vi "test16-LosslessRegisterStatusMultipleTimesNonCSM.vi"(8 "error in (no error)":errorcluster, 11 "TestCase in":refnum<class "testcase-CSMBroadcast.lvclass">) -> (0 "error out":errorcluster, 3 "TestCase out":refnum<class "testcase-CSMBroadcast.lvclass">)   [LabVIEW 2017, in "testcase-CSMBroadcast.lvclass"]
uses:
  testcase-CSMBroadcast.lvclass
  <vilib>/addons/_JKI Toolkits/VI Tester/TestCase.llb/TestCase.lvclass
  src/user.lib/_NEVSTOP/Communicable State Machine(CSM)/Communicable State Machine.lvlib
  CSM/CSM-Testcase.lvlib
  C:/Program Files (x86)/National Instruments/LabVIEW 2017/vi.lib/addons/_JKI Toolkits/VI Tester/TestCase.llb/TestCase.lvclass
panel:
  out "Arguments":string
  out "ModuleName":string
  out "LoopCount":i32
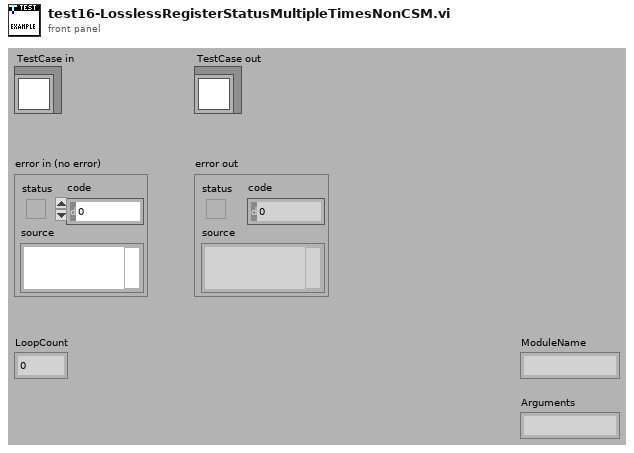
[diagram p1: front panel]
types:
  T1 = cluster{"ModuleName":string, "Status":string, "Arguments":string}
  T2 = cluster{"cluster":cluster{"ModuleName":string, "Status":string, "Arguments":string}, "Counter":u32}
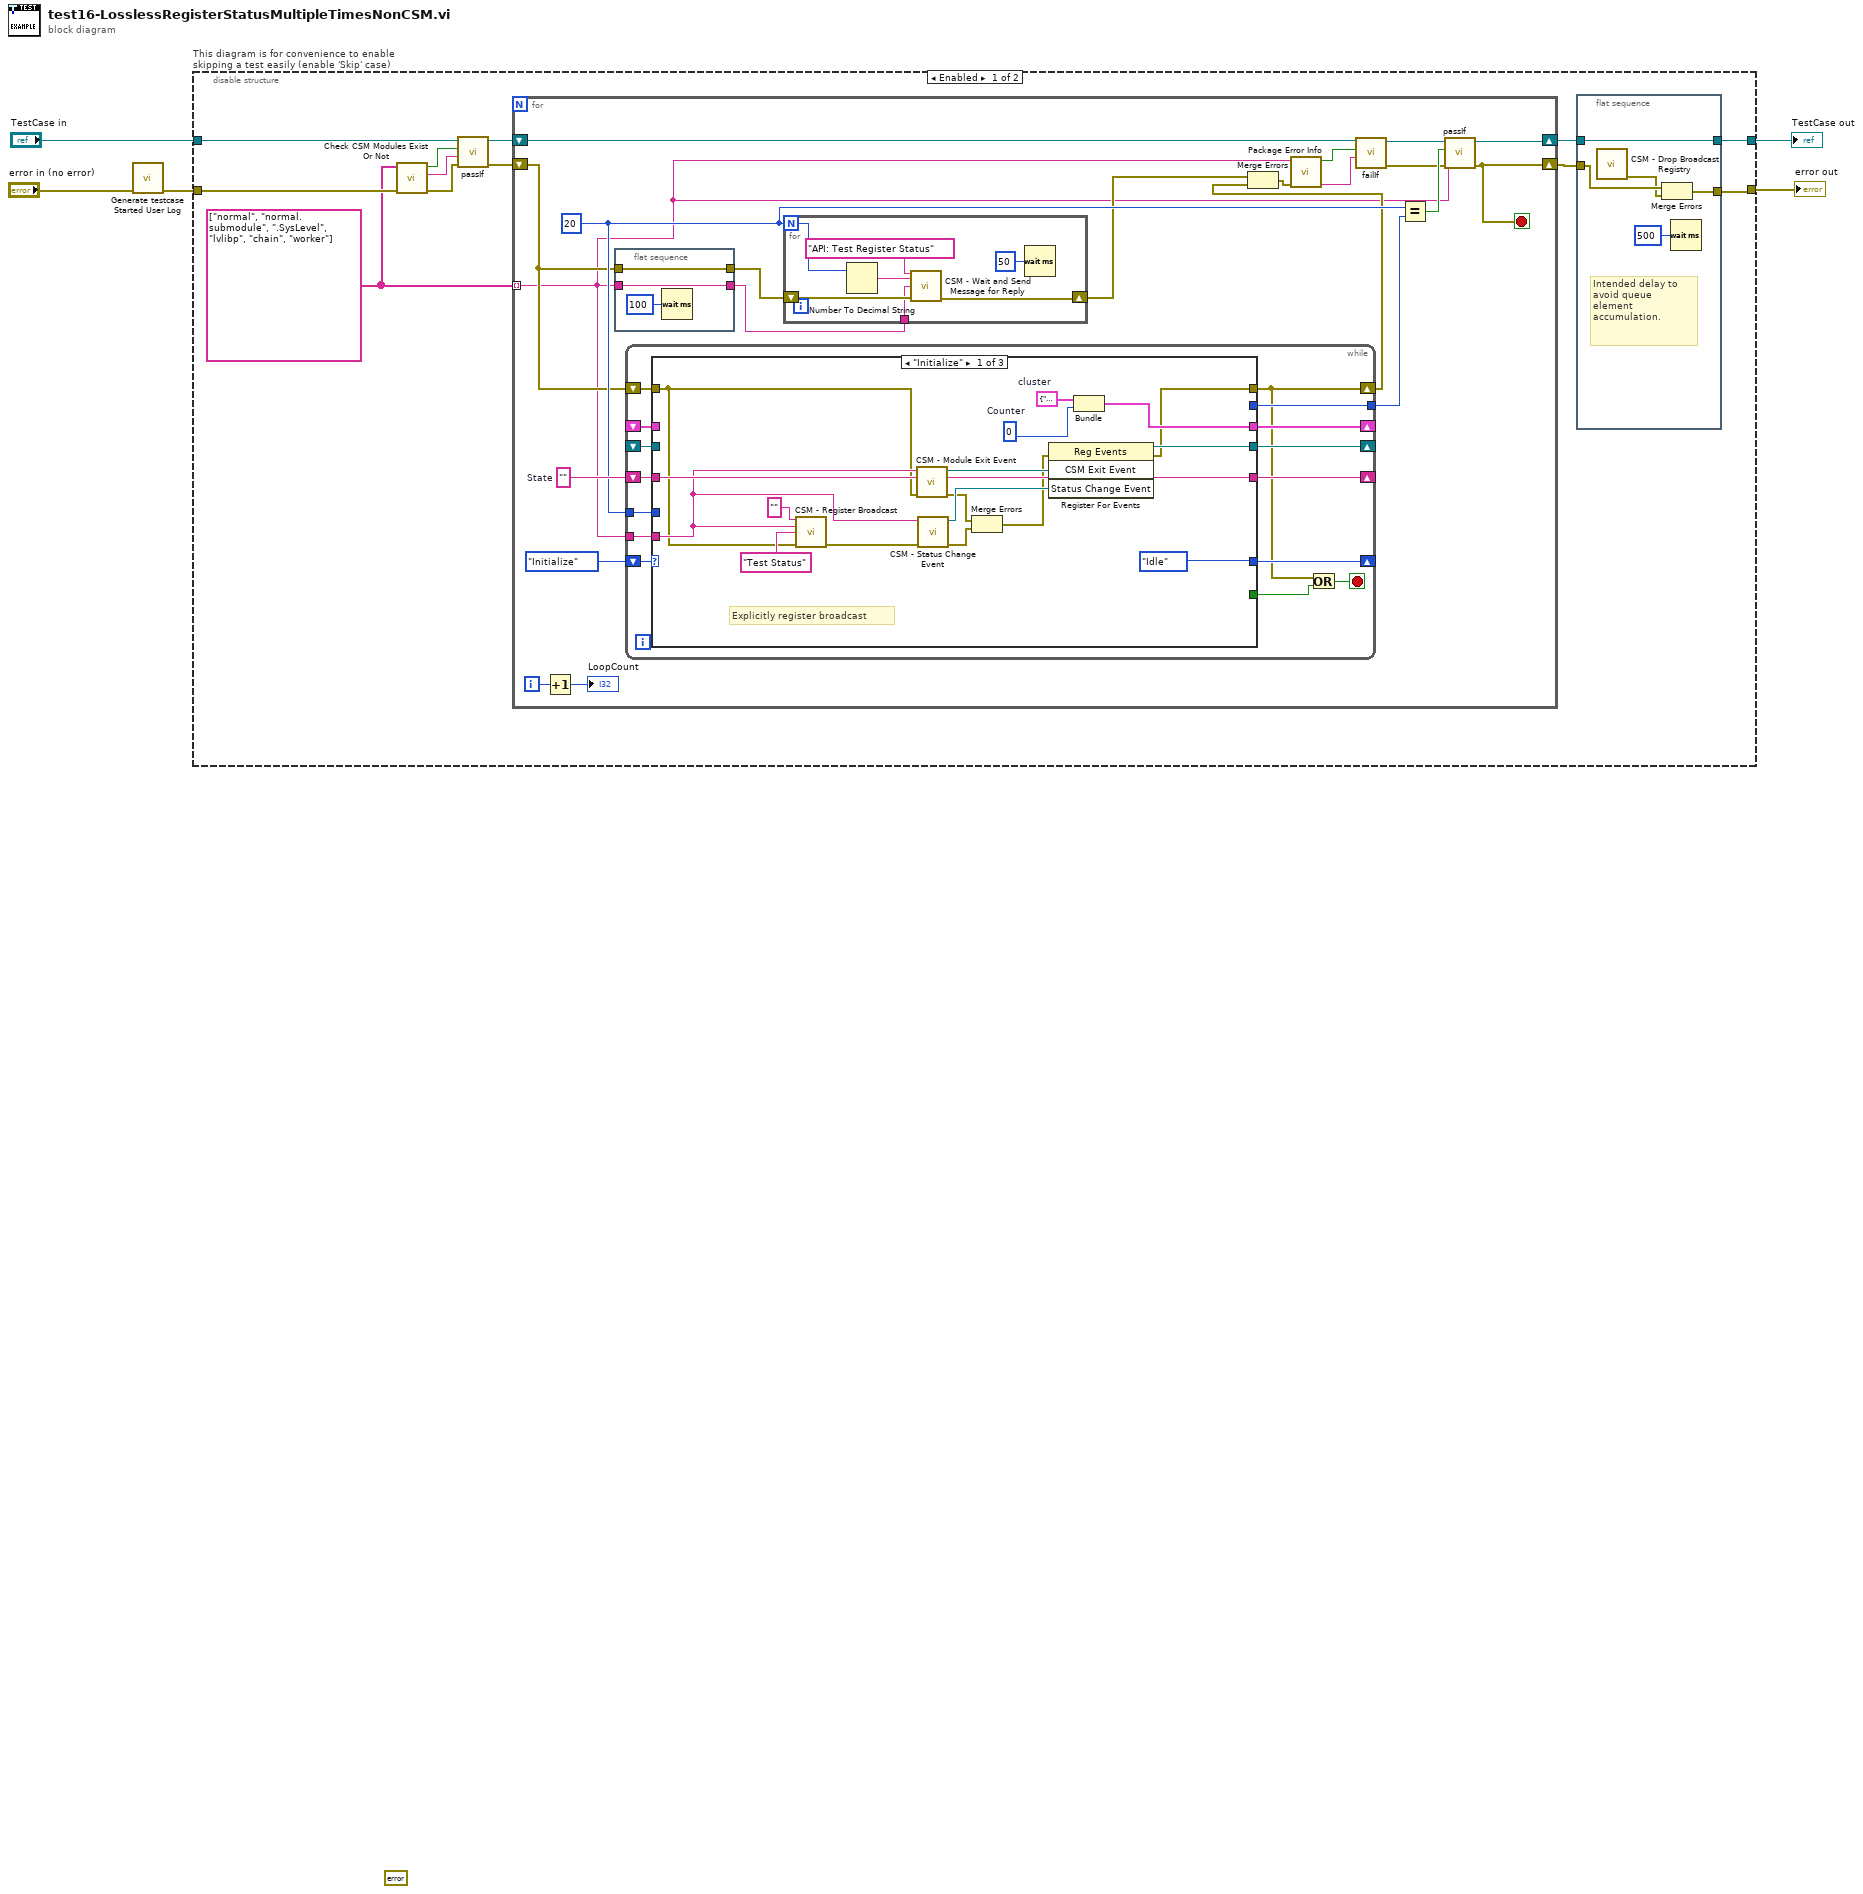
[diagram p0: block diagram]
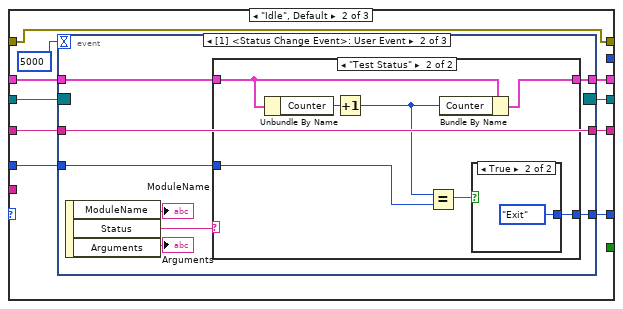
[diagram p2: hidden frame]
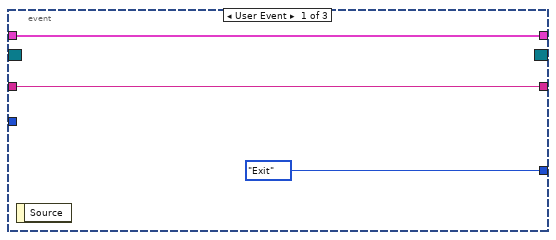
[diagram p3: hidden frame]
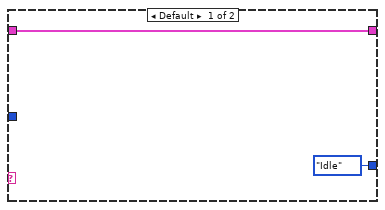
[diagram p4: hidden frame]
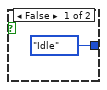
[diagram p5: hidden frame]
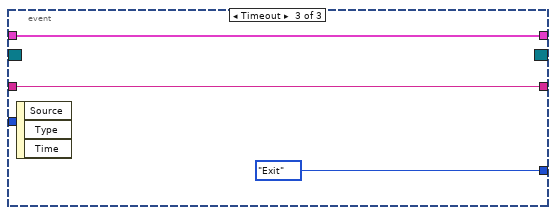
[diagram p6: hidden frame]
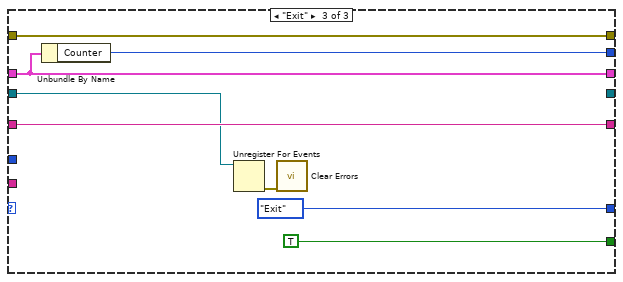
[diagram p7: hidden frame]
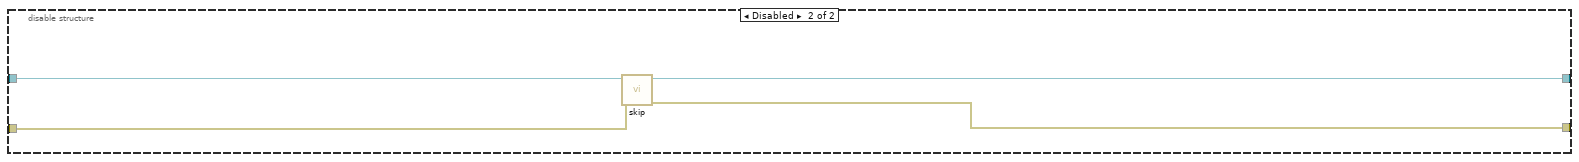
[diagram p8: hidden frame]
diagram:
  (unwired) errorcluster {"status"=FALSE, "code"=0, "source"=""} ("error out")
  n1 = call "Generate testcase Started User Log.vi"("Error In"="error in (no error)") -> ("error out"=w1:errorcluster)  [unwired: 10 in]
  n2 = disable-structure "This diagram is for convenience to enable skipping a test easily (enable 'Skip' case)" shown="Enabled" {
    disable-tunnel: "TestCase in" -> [w12 w132]
    disable-tunnel: [w6 w130] -> w3
    disable-tunnel: [w16 w131] -> w2
    disable-tunnel: w1 -> [w9 w129]
    frame Enabled {
      w8 = string[] ["normal", "normal.submodule", ".SysLevel", "lvlibp", "chain", "worker"]
      n3 = call "Check CSM Modules Exist Or Not.vi"("error in"=w9, "CSM names in"=w8) -> ("error out"=w13:errorcluster, "Debug string"=w14:string, "All Modules Exist?"=w15:bool)  [unwired: 7 in]
      n4 = call-dynamic "passIf.vi"("error in (no error)"=w13, "message (\"\")"=w14, "pass"=w15, "TestCase in"=w12) -> ("error out"=w10:errorcluster, "TestCase out"=w11:refnum<class "testcase-CSMBroadcast.lvclass">)  [unwired: 6 in]
      n5 = for {
        shift-right: [w41] -> w7
        shift-left: w11 -> [w25]
        shift-right: [w38] -> w17
        shift-left: w10 -> [w32]
        tunnel: w8 -> [w26] mode=indexing
        i -> [w40]
        stop <- w38 stop-if-true
        w34 = 20
        w42 = ""  # State
        n6 = Increment(x=w40) -> (x+1=→"LoopCount":i32)
        n7 = flat-sequence {
          tunnel: w26 -> [w53]
          tunnel: [w53] -> w37
          tunnel: w32 -> [w51]
          tunnel: [w51] -> w33
          frame #0 {
            n8 = Wait (ms)(milliseconds to wait=u32 100) -> ()  [unwired: 1 out]
          }
        }
        n9 = while {
          shift-right: [w67] -> _
          shift-left: enum16{"Idle", "Initialize", "Exit"}."Initialize" -> [w68]
          shift-right: [w65] -> _
          shift-left: w42 -> [w66]
          shift-right: [w64] -> _
          shift-left: _ -> [w63]
          shift-right: [w62] -> _
          shift-left: _ -> [w61]
          tunnel: w26 -> [w60]
          tunnel: [w59] -> w36
          tunnel: w34 -> [w58]
          shift-right: [w56] -> w29
          shift-left: w32 -> [w57]
          stop <- w54 stop-if-true
          n10 = case shown="\"Initialize\"" w68 {
            tunnel: [enum16{"Idle", "Initialize", "Exit"}."Idle" w95 enum16{"Idle", "Initialize", "Exit"}."Exit"] -> w67
            tunnel: [_ _ TRUE] -> w55
            tunnel: w66 -> [w84 w93 w126]
            tunnel: [w84 w94 w126] -> w65
            tunnel: [w82 w91 _] -> w64
            tunnel: w63 -> [_ w92 w125]
            tunnel: [w81 w89 w122] -> w62
            tunnel: w61 -> [_ w90 w122]
            tunnel: w60 -> [w73 _ _]
            tunnel: [_ _ w123] -> w59
            tunnel: w58 -> [_ w87 _]
            tunnel: w57 -> [w71 w86 w121]
            tunnel: [w69 w86 w121] -> w56
            frame "Initialize" {
              w76 = u32 0  # Counter
              w79 = T1 {"ModuleName"="", "Status"="", "Arguments"=""}  # cluster
              # "Explicitly register broadcast"
              n11 = call "CSM - Register Broadcast.vi"("CSM Name(Empty for Broadcast Event)"="", "Source CSM Name (* as Default)"=w73, "Trigger"="Test Status" ("State"), "Error In"=w71) -> ("error out"=w72:errorcluster)  [unwired: 10 in, 1 out]
              n12 = call "CSM - Module Exit Event.vi"("Error In"=w71, "Name (\"\" to Use UUID) In"=w73) -> ("error out"=w78:errorcluster, "CSM Exit Event"=w83:refnum<user-event>)  [unwired: 7 in, 1 out]
              n13 = call "CSM - Status Change Event.vi"("Error In"=w72, "CSM Module"=w73) -> ("error out"=w77:errorcluster, "Status Change Event"=w80:refnum<user-event>)  [unwired: 7 in, 1 out]
              n14 = Merge Errors(w78, w77) -> (w70:errorcluster)
              n15 = register-events(error in=w70, w83, w80) -> (reference out=w82:refnum<event-registration>, error out=w69:errorcluster)  [unwired: 1 in]
              n16 = Bundle("cluster"=w79, "Counter"=w76) -> (w81:T2)  [unwired: 1 in]
            }
            frame "Idle", Default {
              n17 = event shown="[1] <Status Change Event>: User Event" {
                selector: w92 -> [_ _ _]
                dyn-events: [_ _ _] -> w91
                timeout: 5000 -> [_ _ _]
                tunnel: [enum16{"Idle", "Initialize", "Exit"}."Exit" w105 enum16{"Idle", "Initialize", "Exit"}."Exit"] -> w95
                tunnel: w93 -> [w98 w106 w120]
                tunnel: [w98 w106 w120] -> w94
                tunnel: w90 -> [w96 w103 w119]
                tunnel: [w96 w104 w119] -> w89
                tunnel: w87 -> [_ w102 _]
                event User Event {
                  n18 = event-data() -> ()  [unwired: 1 in, 1 out]
                }
                event User Event {
                  n19 = event-data() -> ("ModuleName"=→"ModuleName":string, "Status"=w101:string, "Arguments"=→"Arguments":string)  [unwired: 1 in]
                  n20 = case shown="\"Test Status\"" w101 {
                    tunnel: [enum16{"Idle", "Initialize", "Exit"}."Idle" w115] -> w105
                    tunnel: [w108 w114] -> w104
                    tunnel: w103 -> [w108 w113]
                    tunnel: w102 -> [_ w109]
                    frame Default {
                    }
                    frame "Test Status" {
                      n21 = Unbundle By Name(w113) -> ("Counter"=w112:u32)
                      n22 = Increment(x=w112) -> (x+1=w110:u32)
                      n23 = Equal?(x=w110, y=w109) -> (x = y?=w111:bool)
                      n24 = Bundle By Name(cluster=w113, "Counter"=w110) -> (w114:T2)
                      n25 = case shown="True" w111 {
                        tunnel: [enum16{"Idle", "Initialize", "Exit"}."Idle" enum16{"Idle", "Initialize", "Exit"}."Exit"] -> w115
                        frame False {
                        }
                        frame True {
                        }
                      }
                    }
                  }
                }
                event Timeout {
                  n26 = event-data() -> ()  [unwired: 1 in, 3 out]
                }
              }
            }
            frame "Exit" {
              n27 = Unbundle By Name(w122) -> ("Counter"=w123:u32)
              n28 = Unregister For Events(event registration refnum=w125) -> (error out=w124:errorcluster)  [unwired: 1 in]
              n29 = call <vilib>:"Clear Errors.vi"("error in (no error)"=w124) -> ()  [unwired: 5 in, 2 out]
            }
          }
          n30 = Or(x=w56, y=w55) -> (x .or. y?=w54:bool)
        }
        n31 = for {
          N: w34 -> [w48]
          shift-right: [w46] -> w27
          shift-left: w33 -> [w47]
          tunnel: w37 -> [w45]
          n32 = Number To Decimal String(number=w48) -> (decimal integer string=w49:string)  [unwired: 1 in]
          n33 = call "CSM - Wait and Send Message for Reply.vi"("State"="API: Test Register Status", "Arguments (\"\")"=w49, "Target Module"=w45, "Error In (No Error)"=w47) -> ("error out"=w46:errorcluster)  [unwired: 8 in, 3 out]
          n34 = Wait (ms)(milliseconds to wait=u32 50) -> ()  [unwired: 1 out]
        }
        n35 = Merge Errors(w27, w29) -> (w28:errorcluster)
        n36 = call "Package Error Info.vi"("error in"=w28, "String in"=w26) -> ("packed error info out"=w30:string, "error status"=w31:bool)  [unwired: 8 in]
        n37 = call-dynamic "failIf.vi"("message (\"\")"=w30, "fail"=w31, "TestCase in"=w25) -> ("error out"=w23:errorcluster, "TestCase out"=w24:refnum<class "testcase-CSMBroadcast.lvclass">)  [unwired: 7 in]
        n38 = Equal?(x=w34, y=w36) -> (x = y?=w35:bool)
        n39 = call-dynamic "passIf.vi"("error in (no error)"=w23, "message (\"\")"=w26, "pass"=w35, "TestCase in"=w24) -> ("error out"=w38:errorcluster, "TestCase out"=w41:refnum<class "testcase-CSMBroadcast.lvclass">)  [unwired: 6 in]
      }
      n40 = flat-sequence {
        tunnel: w17 -> [w22]
        tunnel: [w21] -> w16
        tunnel: w7 -> [w19]
        tunnel: [w19] -> w6
        frame #0 {
          # "Intended delay to\navoid queue\nelement\naccumulation."
          n41 = call "CSM - Drop Broadcast Registry.vi"() -> ("error out"=w20:errorcluster)  [unwired: 15 in]
          n42 = Merge Errors(w22, w20) -> (w21:errorcluster)
          n43 = Wait (ms)(milliseconds to wait=u32 500) -> ()  [unwired: 1 out]
        }
      }
    }
    frame Disabled {
      # "skip test result while test is under development"
      n44 = call <vilib>:"skip.vi"("error in (no error)"=w129, "TestCase in"=w132) -> ("error out"=w131:errorcluster, "TestCase out"=w130:refnum<class "testcase-CSMBroadcast.lvclass">)  [unwired: 8 in]
    }
  }
  "error out" <- w2
  "TestCase out" <- w3
